vi "Scan Data Save.vi"(8 "error in (no error)":errorcluster, 9 "index":i32=30, 10 "OK and NG":bool, 11 "String In":string="$AGENT.81,C8.C8,S*03") -> (0 "error out":errorcluster)   [LabVIEW 2019]
uses:
  Ctrl/MeasureDisplayTab.ctl
  Ctrl/Table Save.ctl
  LLB/Commonly VI/Main Glb.vi
  LLB/Commonly VI.lvlib
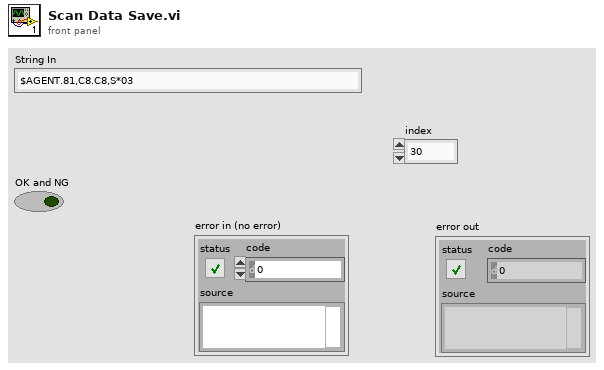
[diagram p1: front panel]
types:
  T1 = typedef "Table Save.ctl" = enum16{"initial", "Add", "Write", "Replace", "Delete", "REad", "RedTable", "Load"}
  T2 = typedef "MeasureDisplayTab.ctl" = enum16{"Tray Barcode", "PCBA BARCODE", "硬體(Tool初始化)", "company(Tool初始化)", "耗電流 uA(電流表)", "電池負載電壓", "晶片ID(Tool FORMAT)", "雷雕ID(TOOl scan、藍芽接收器)", "Format(Tool FORMAT)", "Programe(Tool Programe)", "MAC(藍芽接收器)", "ID(藍芽接收器)", "KPA(藍芽接收器)", "溫度(藍芽接收器)", "SENSOR電池電壓(藍芽接收器)", "RSSI(藍芽接收器)", "SensorType_315(FSK scan)", "FSKsnVol_315(FSK scan)", "FSKscanl_315(FSK scan)", "P_315(FSK scan)", "T_315(FSK scan)", "SensorType_433(ASK scan)", "ASKsnVol_433(ASK scan)", "ASKscan_433(ASK scan)", "P_433(ASK scan)", "T_433(ASK scan)", "測高Data"}
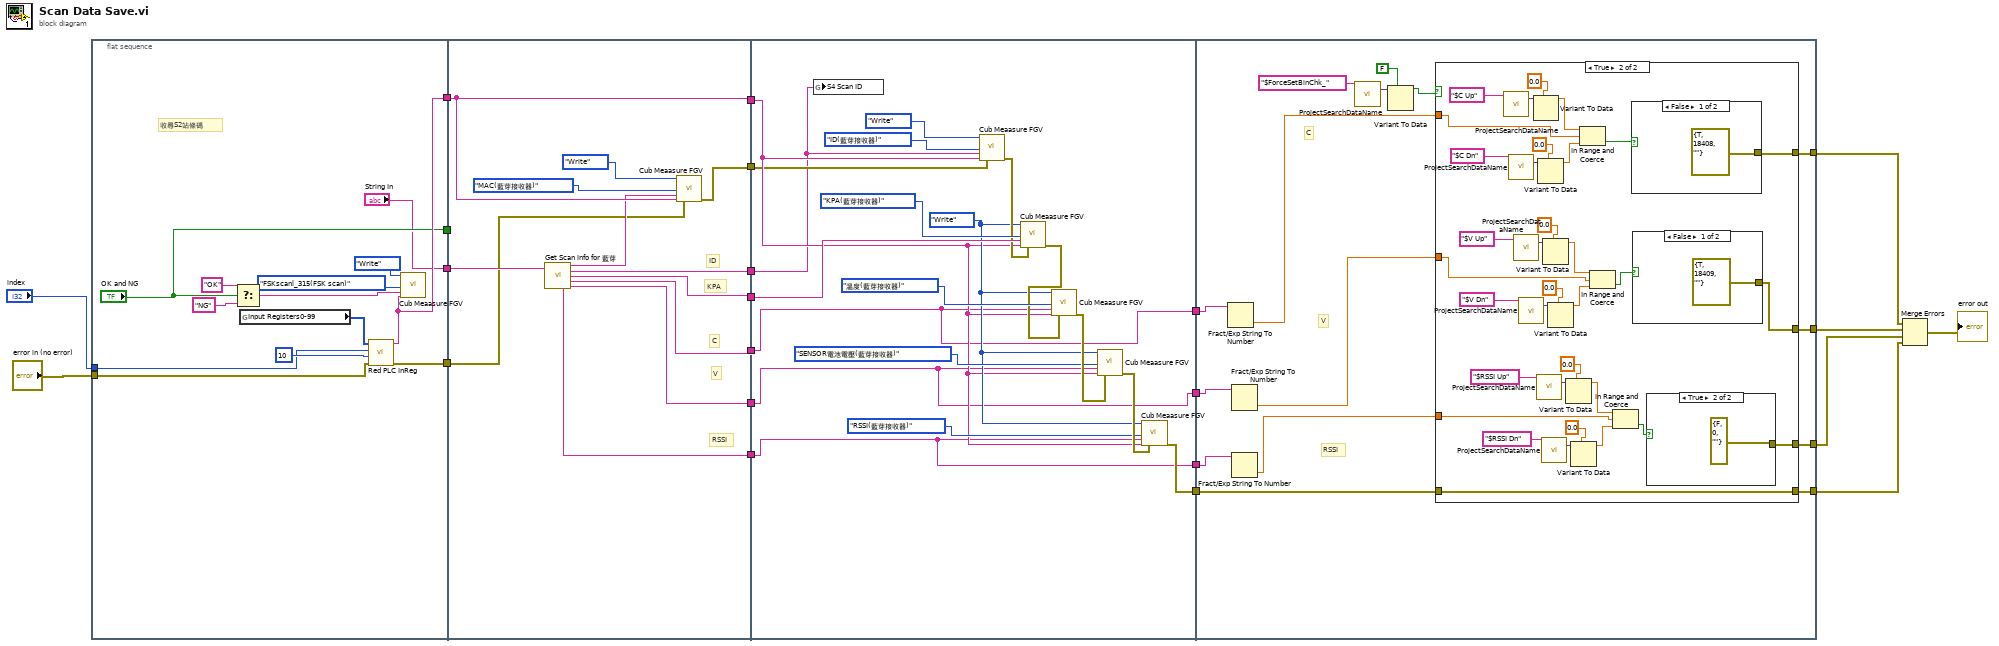
[diagram p0: block diagram]
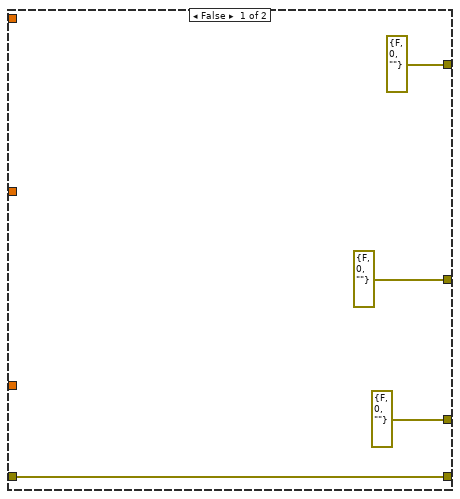
[diagram p2: hidden frame]
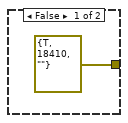
[diagram p3: hidden frame]
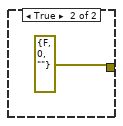
[diagram p4: hidden frame]
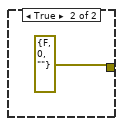
[diagram p5: hidden frame]
diagram:
  n1 = flat-sequence {
    tunnel: [w28] -> w22
    tunnel: ["OK and NG"] -> w20
    tunnel: "error in (no error)" -> [w24]
    tunnel: [w23] -> w18
    tunnel: ["String In"] -> w17
    tunnel: "index" -> [w25]
    tunnel: w22 -> [w47]
    tunnel: [w47] -> w21
    tunnel: w20 -> [_]
    tunnel: w18 -> [w37]
    tunnel: w17 -> [w46]
    tunnel: [w42] -> w15
    tunnel: [w41] -> w14
    tunnel: [w40] -> w13
    tunnel: [w39] -> w12
    tunnel: [w38] -> w11
    tunnel: [w36] -> w10
    tunnel: w21 -> [w54]
    tunnel: w15 -> [w48]
    tunnel: w14 -> [w63]
    tunnel: w13 -> [w51]
    tunnel: w12 -> [w50]
    tunnel: w11 -> [w49]
    tunnel: w10 -> [w53]
    tunnel: [w52] -> w9
    tunnel: [w51] -> w8
    tunnel: [w50] -> w7
    tunnel: [w49] -> w6
    tunnel: w9 -> [w71]
    tunnel: w8 -> [w77]
    tunnel: w7 -> [w76]
    tunnel: w6 -> [w75]
    tunnel: [w70] -> w5
    tunnel: [w69] -> w4
    tunnel: [w68] -> w3
    tunnel: [w67] -> w1
    frame #0 {
      # "收尋S2站條碼"
      n2 = Select(t="OK" ("DataIn"), s="OK and NG", f="NG" ("DataIn")) -> (s? t:f=w35:string)
      n3 = global read "Main Glb.vi" "Input Registers0-99"() -> (w29:u16[])
      n4 = call "Red PLC InReg.vi"("error in (no error)"=w24, "length"=10, "index"=w25, "Input Registers Arr"=w29) -> ("error out"=w23:errorcluster, "Rad In Reg"=w28:string)  [unwired: 6 in]
      n5 = call "Cub Meaasure FGV.vi"("Action"=Table_Save."Write" ("Enum"), "Save Index"=MeasureDisplayTab."FSKscanl_315(FSK scan)", "DataIn"=w35, "SN"=w28) -> ()  [unwired: 8 in, 8 out]
    }
    frame #1 {
      # "RSSI"
      # "V"
      # "C"
      # "KPA"
      # "ID"
      n6 = call "Get Scan Info for 藍芽.vi"("String Input"=w46) -> ("MAC"=w43:string, "ID"=w42:string, "KPA"=w41:string, "C"=w40:string, "RSSI"=w38:string, "V"=w39:string)  [unwired: 9 in]
      n7 = call "Cub Meaasure FGV.vi"("Action"=Table_Save."Write" ("Enum"), "Save Index"=MeasureDisplayTab."MAC(藍芽接收器)", "DataIn"=w43, "SN"=w47, "error in (no error)"=w37) -> ("error out"=w36:errorcluster)  [unwired: 7 in, 7 out]
    }
    frame #2 {
      w56 = Table_Save."Write" ("Enum")
      n8 = global write "Main Glb.vi" "S4 Scan ID"(w48) -> ()
      n9 = call "Cub Meaasure FGV.vi"("Action"=Table_Save."Write" ("Enum"), "Save Index"=MeasureDisplayTab."ID(藍芽接收器)", "DataIn"=w48, "SN"=w54, "error in (no error)"=w53) -> ("error out"=w62:errorcluster)  [unwired: 7 in, 7 out]
      n10 = call "Cub Meaasure FGV.vi"("Action"=w56, "Save Index"=MeasureDisplayTab."KPA(藍芽接收器)", "DataIn"=w63, "SN"=w54, "error in (no error)"=w62) -> ("error out"=w60:errorcluster)  [unwired: 7 in, 7 out]
      n11 = call "Cub Meaasure FGV.vi"("Action"=w56, "Save Index"=MeasureDisplayTab."溫度(藍芽接收器)", "DataIn"=w51, "SN"=w54, "error in (no error)"=w60) -> ("error out"=w59:errorcluster)  [unwired: 7 in, 7 out]
      n12 = call "Cub Meaasure FGV.vi"("Action"=w56, "Save Index"=MeasureDisplayTab."SENSOR電池電壓(藍芽接收器)", "DataIn"=w50, "SN"=w54, "error in (no error)"=w59) -> ("error out"=w57:errorcluster)  [unwired: 7 in, 7 out]
      n13 = call "Cub Meaasure FGV.vi"("Action"=w56, "Save Index"=MeasureDisplayTab."RSSI(藍芽接收器)", "DataIn"=w49, "SN"=w54, "error in (no error)"=w57) -> ("error out"=w52:errorcluster)  [unwired: 7 in, 7 out]
    }
    frame #3 {
      # "RSSI"
      # "V"
      # "C"
      n14 = Fract/Exp String To Number(string=w77) -> (number=w74:dbl)  [unwired: 3 in, 1 out]
      n15 = Fract/Exp String To Number(string=w76) -> (number=w73:dbl)  [unwired: 3 in, 1 out]
      n16 = Fract/Exp String To Number(string=w75) -> (number=w72:dbl)  [unwired: 3 in, 1 out]
      n17 = call "ProjectSearchDataName.vi"("element"="$ForceSetBinChk_") -> ("variant"=w80:variant)  [unwired: 7 in, 3 out]
      n18 = Variant To Data(type=FALSE, Variant=w80) -> (data=w81:bool)  [unwired: 1 in, 1 out]
      n19 = case shown="True" w81 {
        tunnel: w74 -> [_ w103]
        tunnel: w73 -> [_ w102]
        tunnel: w72 -> [_ w93]
        tunnel: w71 -> [w82 w86]
        tunnel: [errorcluster {"status"=FALSE, "code"=0, "source"=""} ("error out") w92] -> w70
        tunnel: [errorcluster {"status"=FALSE, "code"=0, "source"=""} ("error out") w91] -> w69
        tunnel: [errorcluster {"status"=FALSE, "code"=0, "source"=""} ("error out") w87] -> w68
        tunnel: [w82 w86] -> w67
        frame False {
        }
        frame True {
          n20 = call "ProjectSearchDataName.vi"("element"="$C Up") -> ("variant"=w118:variant)  [unwired: 7 in, 3 out]
          n21 = call "ProjectSearchDataName.vi"("element"="$C Dn") -> ("variant"=w117:variant)  [unwired: 7 in, 3 out]
          n22 = call "ProjectSearchDataName.vi"("element"="$V Up") -> ("variant"=w105:variant)  [unwired: 7 in, 3 out]
          n23 = call "ProjectSearchDataName.vi"("element"="$V Dn") -> ("variant"=w106:variant)  [unwired: 7 in, 3 out]
          n24 = Variant To Data(type=0.0, Variant=w118) -> (data=w115:dbl)  [unwired: 1 in, 1 out]
          n25 = call "ProjectSearchDataName.vi"("element"="$RSSI Up") -> ("variant"=w100:variant)  [unwired: 7 in, 3 out]
          n26 = Variant To Data(type=0.0, Variant=w117) -> (data=w114:dbl)  [unwired: 1 in, 1 out]
          n27 = call "ProjectSearchDataName.vi"("element"="$RSSI Dn") -> ("variant"=w99:variant)  [unwired: 7 in, 3 out]
          n28 = Variant To Data(type=0.0, Variant=w105) -> (data=w108:dbl)  [unwired: 1 in, 1 out]
          n29 = Variant To Data(type=0.0, Variant=w106) -> (data=w109:dbl)  [unwired: 1 in, 1 out]
          n30 = Variant To Data(type=0.0, Variant=w100) -> (data=w97:dbl)  [unwired: 1 in, 1 out]
          n31 = Variant To Data(type=0.0, Variant=w99) -> (data=w96:dbl)  [unwired: 1 in, 1 out]
          n32 = In Range and Coerce(upper limit=w115, x=w103, lower limit=w114) -> (In Range?=w90:bool)  [unwired: 1 out]
          n33 = In Range and Coerce(upper limit=w108, x=w102, lower limit=w109) -> (In Range?=w89:bool)  [unwired: 1 out]
          n34 = In Range and Coerce(upper limit=w97, x=w93, lower limit=w96) -> (In Range?=w88:bool)  [unwired: 1 out]
          n35 = case shown="False" w90 {
            tunnel: [errorcluster {"status"=TRUE, "code"=18408, "source"=""} ("error out") errorcluster {"status"=FALSE, "code"=0, "source"=""} ("error out")] -> w92
            frame False {
            }
            frame True {
            }
          }
          n36 = case shown="False" w89 {
            tunnel: [errorcluster {"status"=TRUE, "code"=18409, "source"=""} ("error out") errorcluster {"status"=FALSE, "code"=0, "source"=""} ("error out")] -> w91
            frame False {
            }
            frame True {
            }
          }
          n37 = case shown="True" w88 {
            tunnel: [errorcluster {"status"=TRUE, "code"=18410, "source"=""} ("error out") errorcluster {"status"=FALSE, "code"=0, "source"=""} ("error out")] -> w87
            frame False {
            }
            frame True {
            }
          }
        }
      }
    }
  }
  n38 = Merge Errors(w5, w4, w3, w1) -> (→"error out":errorcluster)
